vi "LaserScan2ROSMsg.vi"(10 "LaserScan":T1, 11 "msg in":string) -> (3 "msg out":string)   [LabVIEW 2014]
uses:
  LaserScan.ctl
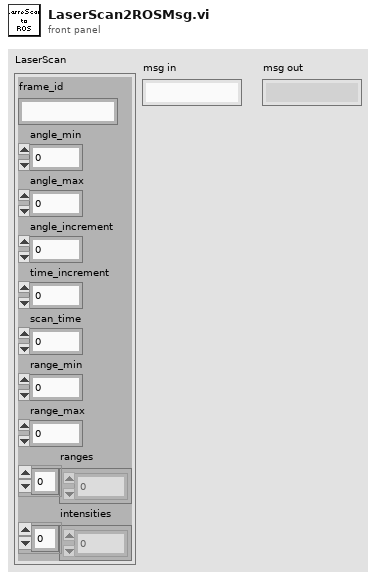
[diagram p1: front panel]
types:
  T1 = typedef "LaserScan.ctl" = cluster{"frame_id":string, "angle_min":dbl, "angle_max":dbl, "angle_increment":dbl, "time_increment":dbl, "scan_time":dbl, "range_min":dbl, "range_max":dbl, "ranges":dbl[], "intensities":dbl[]}
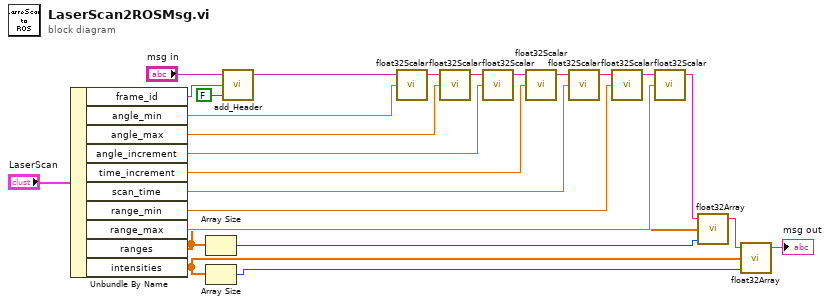
[diagram p0: block diagram]
diagram:
  n1 = Unbundle By Name("LaserScan") -> ("frame_id"=w24:string, "angle_min"=w22:dbl, "angle_max"=w21:dbl, "angle_increment"=w20:dbl, "time_increment"=w19:dbl, "scan_time"=w18:dbl, "range_min"=w17:dbl, "range_max"=w16:dbl, "ranges"=w14:dbl[], "intensities"=w10:dbl[])
  n2 = Array Size(array=w14) -> (size(s)=w13:i32)
  n3 = Array Size(array=w10) -> (size(s)=w2:i32)
  n4 = call <userlib>:"add_Header.vi"("reset seq?"=FALSE, "frame_id"=w24, "msg in"="msg in") -> ("msg out"=w1:string)  [unwired: 2 in]
  n5 = call <userlib>:"float32Scalar.vi"("Numeric"=w22, "msg in"=w1) -> ("msg out"=w9:string)  [unwired: 3 in]
  n6 = call <userlib>:"float32Scalar.vi"("Numeric"=w21, "msg in"=w9) -> ("msg out"=w8:string)  [unwired: 3 in]
  n7 = call <userlib>:"float32Scalar.vi"("Numeric"=w20, "msg in"=w8) -> ("msg out"=w7:string)  [unwired: 3 in]
  n8 = call <userlib>:"float32Scalar.vi"("Numeric"=w19, "msg in"=w7) -> ("msg out"=w6:string)  [unwired: 3 in]
  n9 = call <userlib>:"float32Scalar.vi"("Numeric"=w18, "msg in"=w6) -> ("msg out"=w5:string)  [unwired: 3 in]
  n10 = call <userlib>:"float32Scalar.vi"("Numeric"=w17, "msg in"=w5) -> ("msg out"=w4:string)  [unwired: 3 in]
  n11 = call <userlib>:"float32Scalar.vi"("Numeric"=w16, "msg in"=w4) -> ("msg out"=w15:string)  [unwired: 3 in]
  n12 = call <userlib>:"float32Array.vi"("Array Length"=w13, "Array"=w14, "msg in"=w15) -> ("msg out"=w3:string)  [unwired: 2 in]
  n13 = call <userlib>:"float32Array.vi"("Array Length"=w2, "Array"=w10, "msg in"=w3) -> ("msg out"=→"msg out":string)  [unwired: 2 in]
